vi "MoveContactSeparation.vi"() -> ()   [LabVIEW 2015]
uses:
  Interface.ctl
panel:
  in  "Interface":T1
  in  "contact move?":bool
  out "error code":i32
  out "StringOutputArray":string[](array[string])
  out "Response":string
  in  "VISA Resource":refnum<visa-resource-name>="GPIB0::13::INSTR"
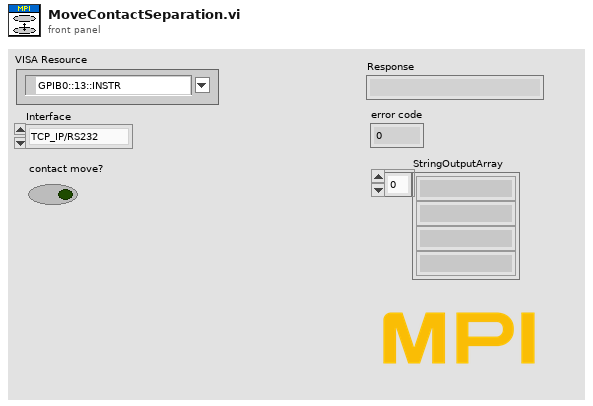
[diagram p1: front panel]
types:
  T1 = typedef "Interface.ctl" = enum16{"TCP_IP/RS232", "GPIB"}
  T2 = enum16{"EndOfLine", "LineFeed", "CarriageReturn"}
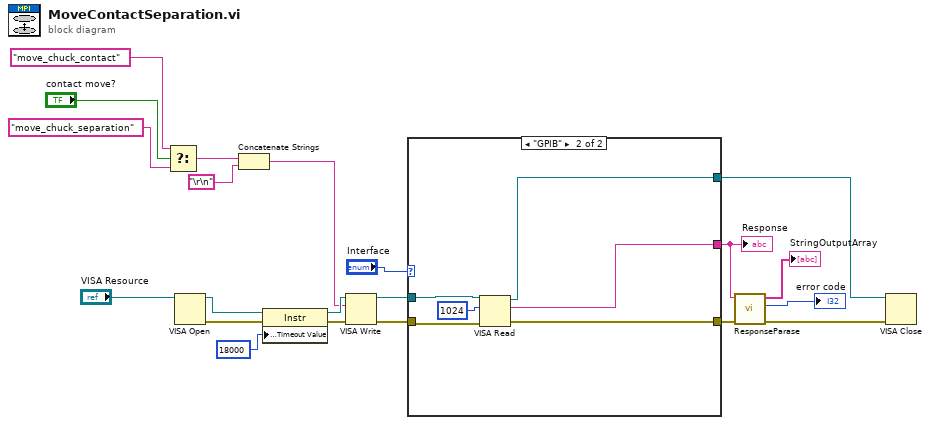
[diagram p0: block diagram]
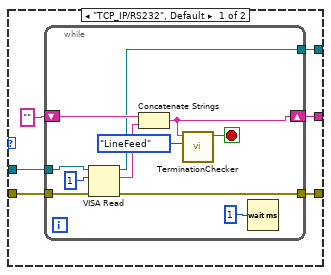
[diagram p2: hidden frame]
diagram:
  n1 = Select(t="move_chuck_contact", s="contact move?", f="move_chuck_separation") -> (s? t:f=w9:string)
  n2 = VISA Open(VISA resource name="VISA Resource") -> (VISA resource name=w19:refnum<visa-resource-name>, error out=w18:errorcluster)  [unwired: 1 in, 3 out]
  n3 = Concatenate Strings(w9, "\r\n") -> (w15:string)
  n4 = property class="Instr"(reference=w19, error in=w18, "General Settings:Timeout Value"=u32 18000) -> (reference out=w17:refnum<visa-resource-name>, error out=w16:errorcluster)
  n5 = VISA Write(VISA resource name=w17, write buffer=w15, error in (no error)=w16) -> (VISA resource name out=w14:refnum<visa-resource-name>, error out=w13:errorcluster)  [unwired: 1 out]
  n6 = case shown="\"GPIB\"" "Interface" {
    tunnel: w14 -> [w27 w42]
    tunnel: w13 -> [w26 w43]
    tunnel: [w24 w39] -> w12
    tunnel: [w23 w41] -> w6
    tunnel: [w22 w40] -> w5
    frame "TCP_IP/RS232", Default {
      n7 = while {
        tunnel: w27 -> [w38]
        tunnel: w26 -> [w37]
        shift-right: [w31] -> w24
        shift-left: "" -> [w35]
        tunnel: [w29] -> w22
        tunnel: [w28] -> w23
        stop <- w33 stop-if-true
        n8 = VISA Read(VISA resource name=w38, byte count=u32 1, error in (no error)=w37) -> (VISA resource name out=w29:refnum<visa-resource-name>, read buffer=w34:string, error out=w28:errorcluster)  [unwired: 1 out]
        n9 = Concatenate Strings(w35, w34) -> (w31:string)
        n10 = call "TerminationChecker.vi"("Type"=T2."LineFeed", "input string"=w31) -> ("Ret"=w33:bool)  [unwired: 9 in]
        n11 = Wait (ms)(milliseconds to wait=u32 1) -> ()  [unwired: 1 out]
      }
    }
    frame "GPIB" {
      n12 = VISA Read(VISA resource name=w42, byte count=u32 1024, error in (no error)=w43) -> (VISA resource name out=w40:refnum<visa-resource-name>, read buffer=w39:string, error out=w41:errorcluster)  [unwired: 1 out]
    }
  }
  "Response" <- w12
  n13 = call "ResponseParase.vi"("error in (no error)"=w6, "input string"=w12) -> ("error out"=w2:errorcluster, "error code"=→"error code":i32, "OutputArray"=→"StringOutputArray":string[])  [unwired: 7 in]
  n14 = VISA Close(VISA resource name=w5, error in (no error)=w2) -> ()  [unwired: 1 out]
